vi "Test Sender field Correct on Receive Requrest Message.vi"(8 "error in (no error)":errorcluster, 11 "Test Case In":refnum<class "Debugger Test.lvclass">) -> (0 "error out":errorcluster, 3 "Test Case Out":refnum<class "Debugger Test.lvclass">)   [LabVIEW 2020, in "Debugger Test.lvclass"]
uses:
  Debugger Test.lvclass
  Debugger Test.lvclass/Debugger Test.ctl
  01074fa8-ee8a-411d-bc8b-fc92c4f90959.vi
  source/Process/Debug Process.lvclass
  source/Debugger/Debugger.lvclass
  source/Debug Data/Debug Data.lvclass
  source/Debug Data/Raw Debug Data.ctl
  C:/Users/anton/Documents/GitHub/triarc-debugger/source/Process/Debug Process.lvclass
  C:/Users/anton/Documents/GitHub/triarc-debugger/source/Debugger/Debugger.lvclass
  C:/Users/anton/Documents/GitHub/triarc-debugger/source/Debug Data Event/Debug Data Listener.lvclass
  <vilib>/Astemes/Triarc Framework/Broadcast Event Helpers/Broadcast Event Helpers.lvlib
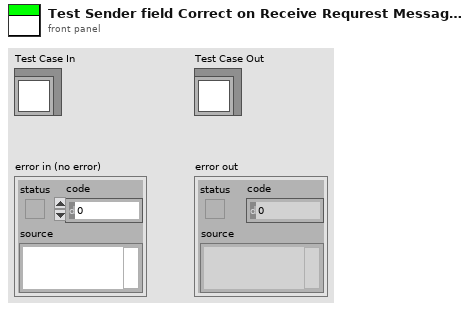
[diagram p1: front panel]
types:
  T1 = typedef "Debug Data.lvclass/Raw Debug Data.ctl" = cluster{"Action":string, "Call Chain":string, "Process":string, "Message":string, "Message Data":variant, "Time":dbl}
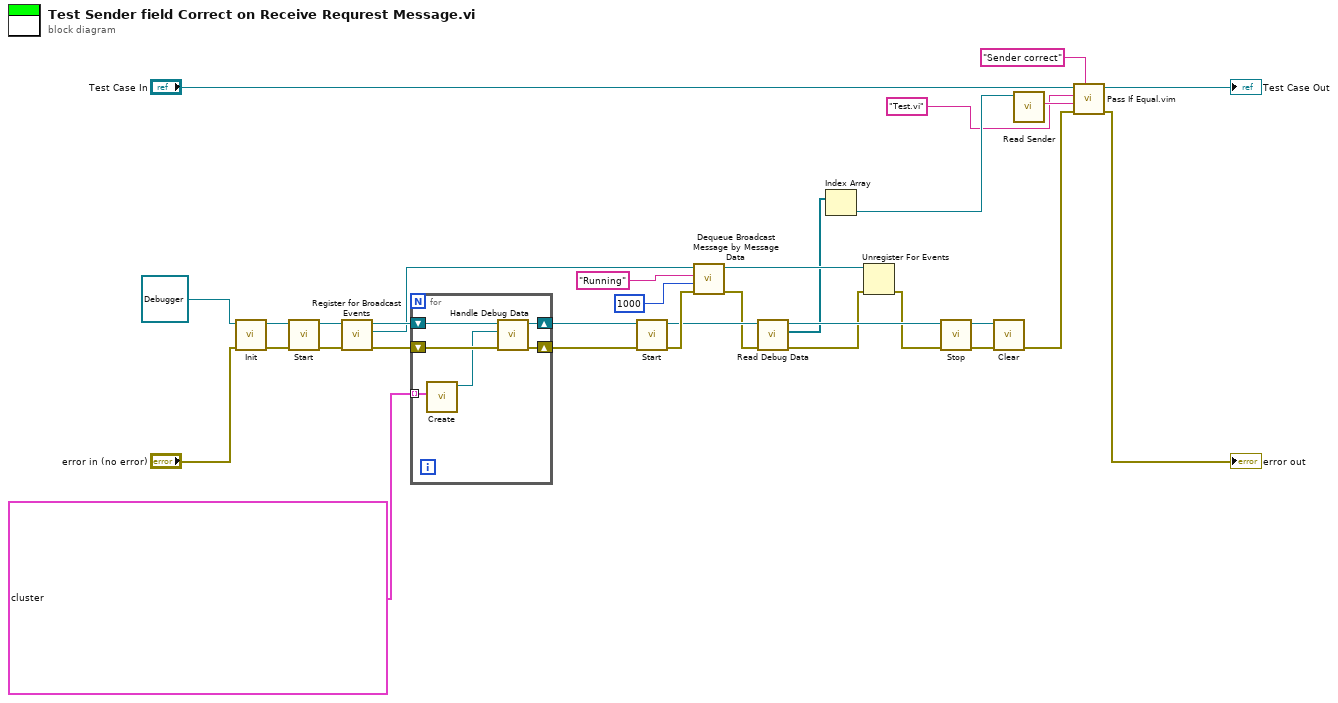
[diagram p0: block diagram]
diagram:
  n1 = call-dynamic "Init.vi"("error in (no error)"="error in (no error)", "Process In"=refnum<class "Debugger.lvclass"> refnum ("Debug Data Event In 2")) -> ("error out"=w28:errorcluster, "Process Out"=w29:refnum<class "Debugger.lvclass">)  [unwired: 8 in]
  n2 = call "Start.vi"("error in (no error)"=w28, "Process In"=w29) -> ("error out"=w26:errorcluster, "Process Out"=w27:refnum<class "Debugger.lvclass">)  [unwired: 7 in, 1 out]
  n3 = call "Register for Broadcast Events.vi"("error in (no error)"=w26, "Process In"=w27) -> ("error out"=w25:errorcluster, "Event Registration Refnum Out"=w7:refnum<event-registration>, "Process Out"=w20:refnum<class "Debugger.lvclass">)  [unwired: 7 in]
  n4 = for {
    shift-right: [w36] -> w24
    shift-left: w25 -> [w38]
    shift-right: [w37] -> w11
    shift-left: w20 -> [w35]
    tunnel: T1[] [{"Action"="Request", "Call Chain"="Test.vi:123456", "Process"="Process 1", "Message"="Init", "Message Data"=variant, "Time"=0.0}, {"Action"="Receive", "Call Chain"="TF.lvlib:Process.lvclass:Handle Messages.vi:1960001", "Process"="Process 1", "Message"="Init", "Message Data"=variant, "Time"=0.0}] ("Debug Data Cluster") -> [w34] mode=indexing
    n5 = call "Create.vi"("Debug Data Cluster"=w34) -> ("Debug Data out"=w33:refnum<class "Debug Data.lvclass">)  [unwired: 9 in, 1 out]
    n6 = call-dynamic "Handle Debug Data.vi"("error in (no error)"=w38, "Debug Data.lvclass"=w33, "Debug Data Event In"=w35) -> ("error out"=w36:errorcluster, "Debug Data Event Out"=w37:refnum<class "Debugger.lvclass">)  [unwired: 7 in]
  }
  n7 = call "Start.vi"("error in (no error)"=w24, "Process In"=w11) -> ("error out"=w12:errorcluster, "Process Out"=w10:refnum<class "Debugger.lvclass">)  [unwired: 7 in, 1 out]
  n8 = call <vilib>:"Dequeue Broadcast Message by Message Data.vi"("error in (no error)"=w12, "Timeout (-1)"=1000, "Message Data"="Running", "Event Registration Refnum"=w7) -> ("error out"=w8:errorcluster, "Event Registration Refnum Out"=w6:refnum<event-registration>)  [unwired: 3 in, 3 out]
  n9 = call "Read Debug Data.vi"("error in (no error)"=w8, "Debugger In"=w10) -> ("error out"=w15:errorcluster, "Data Log"=w3:refnum<class "Debug Data.lvclass">[], "Debugger Out"=w23:refnum<class "Debugger.lvclass">)  [unwired: 7 in]
  n10 = Index Array(array=w3) -> (element=w2:refnum<class "Debug Data.lvclass">)  [unwired: 1 in]
  n11 = Unregister For Events(event registration refnum=w6, error in=w15) -> (error out=w14:errorcluster)
  n12 = call "Stop.vi"("error in (no error)"=w14, "Process In"=w23) -> ("error out"=w21:errorcluster, "Process Out"=w22:refnum<class "Debugger.lvclass">)  [unwired: 7 in, 1 out]
  n13 = call-dynamic "Clear.vi"("error in (no error)"=w21, "Process In"=w22) -> ("error out"=w17:errorcluster)  [unwired: 9 in]
  n14 = call "Read Sender.vi"("Debug Data In"=w2) -> ("Sender"=w9:string)  [unwired: 9 in, 1 out]
  n15 = call "Pass If Equal.vim"("Description"="Sender correct", "error in (no error)"=w17, "Actual"=w9, "Expected"="Test.vi", "LUnit Test Case In"="Test Case In") -> ("error out"=→"error out":errorcluster, "LUnit Test Case Out"=→"Test Case Out":refnum<class "Debugger Test.lvclass">)  [unwired: 5 in]
